vi "Item Info From Tree.vi"(8 "error in":errorcluster, 11 "XML in":string) -> (0 "error out":errorcluster, 2 "Item Info":T1[](array[typedef]), 3 "XML out":string)   [LabVIEW 2020]
uses:
  <vilib>/addons/analyzer/_vianuishared.llb/VIAnUI Item Info.ctl
  <vilib>/addons/analyzer/_vianuishared.llb/VIAnUI Path Type.ctl
  <vilib>/addons/analyzer/_vianuishared.llb/VIAnUI CFG File Info Global.vi
  <vilib>/addons/analyzer/XML Parsing/NI_VIAn_XML Parsing.lvlib
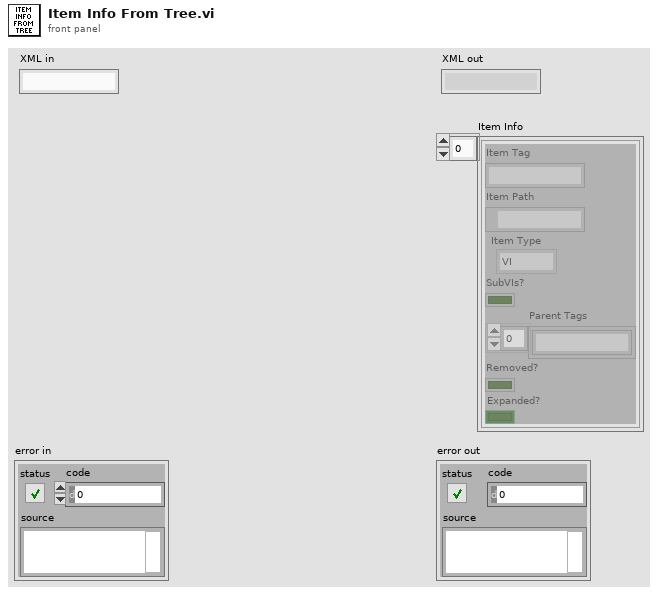
[diagram p1: front panel]
types:
  T1 = typedef "VIAnUI Item Info.ctl" = cluster{"Item Tag":string, "Item Path":path, "Item Type":T2, "SubVIs?":bool, "Parent Tags":string[], "Removed?":bool, "Expanded?":bool}
  T2 = typedef "VIAnUI Path Type.ctl" = enum16{"VI", "LLB", "Folder", "Invalid", "ProjItem"}
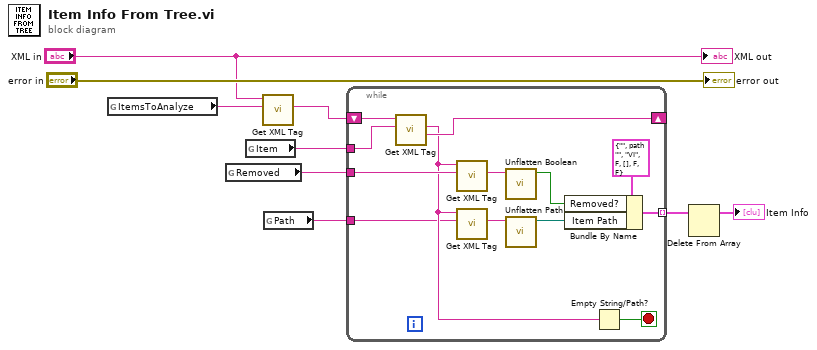
[diagram p0: block diagram]
diagram:
  n1 = global read "VIAnUI CFG File Info Global.vi" "ItemsToAnalyze"() -> (w2:string)
  n2 = global read "VIAnUI CFG File Info Global.vi" "Removed"() -> (w6:string)
  n3 = global read "VIAnUI CFG File Info Global.vi" "Item"() -> (w7:string)
  n4 = call <vilib>:"Get XML Tag.vi"("Tag name"=w2, "XML String in"="XML in") -> ("Tag value"=w9:string)  [unwired: 5 in, 4 out]
  n5 = global read "VIAnUI CFG File Info Global.vi" "Path"() -> (w5:string)
  n6 = while {
    tunnel: [w13] -> w8 mode=indexing
    shift-right: [w21] -> _
    shift-left: w9 -> [w22]
    tunnel: w7 -> [w20]
    tunnel: w6 -> [w18]
    tunnel: w5 -> [w16]
    stop <- w19 stop-if-true
    n7 = call <vilib>:"Get XML Tag.vi"("Tag name"=w20, "XML String in"=w22) -> ("Remaining string"=w21:string, "Tag value"=w17:string)  [unwired: 5 in, 3 out]
    n8 = call <vilib>:"Get XML Tag.vi"("Tag name"=w18, "XML String in"=w17) -> ("Tag value"=w11:string)  [unwired: 5 in, 4 out]
    n9 = call <vilib>:"Get XML Tag.vi"("Tag name"=w16, "XML String in"=w17) -> ("Tag value"=w15:string)  [unwired: 5 in, 4 out]
    n10 = call <vilib>:"Unflatten Boolean.vi"("Tag value"=w11) -> ("Boolean"=w10:bool)  [unwired: 10 in]
    n11 = call <vilib>:"Unflatten Path.vi"("Tag value"=w15) -> ("Path"=w12:path)  [unwired: 10 in]
    n12 = Bundle By Name(cluster=T1 {"Item Tag"="", "Item Path"=path "", "Item Type"=enum."VI", "SubVIs?"=FALSE, "Parent Tags"=[], "Removed?"=FALSE, "Expanded?"=FALSE} ("Item Info"), "Removed?"=w10, "Item Path"=w12) -> (w13:T1)
    n13 = Empty String/Path?(string/path=w17) -> (empty?=w19:bool)
  }
  n14 = Delete From Array(array=w8) -> (array with subset deleted=→"Item Info":T1[])  [unwired: 2 in, 1 out]
  "error out" <- "error in"
  "XML out" <- "XML in"
